vi "fpga_Lowpass filter (P Class_50Hz).vi"(0 "input data":fxp<+/-,24,1>, 1 "reset":bool, 9 "input valid":bool) -> (4 "output data":fxp<+/-,24,2>, 10 "output valid":bool, 14 "ready for input":bool)   [LabVIEW 2013, in "NI_EP_PMU_FPGA.lvlib"]
doc: "----------------------\n\nThis filter is configured as follows:\n\n<b>Filter Configuration</b>\nType: Multirate - Decimation\nStructure: Polyphase FIR\nFactor: 25\n\n<b>Input Data Type</b>\nType: fixed-point <±,24,1> [-1.000000E+0,9.999999E-1]:1.192093E-7\n\n<b>Output Data Type</b>\nType: fixed-point <±,24,2> [-2.000000E+0,2.000000E+0]:2.384186E-7\nRounding mode: Truncate\nOverflow mode: Saturate\n\n<b>Implementation</b>\nNumber of channels: 1\nMaximum input sampling rate per channel @ 40MHz: 8MHz\nGain processing: On Host\nMethod: Multiply-Accumulate\nNumber of multiply pipeline stages: 1\nMultiply register in: False\nState memory: Look-Up Table\nCoefficient memory: Block Memory\n\n<b>Execution Mode</b>\nInside single-cycle Timed Loop\nThroughput: 5 cycles/sample\n\n<b>Estimated Resources</b>\nNumber of multiply-accumulate units: 1\nMultiply operation: I24.1 x I16.-4 => I44.1"
uses:
  <vilib>/addons/Electrical Power/PMU/NI_EP_PMU_FPGA.lvlib
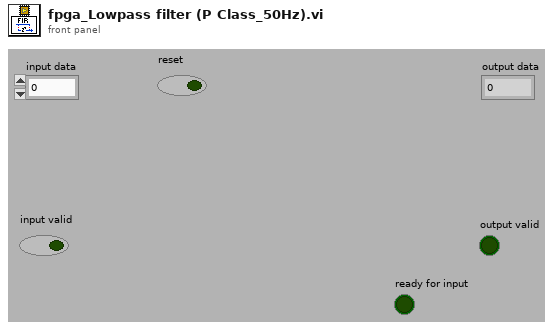
[diagram p1: front panel]
types:
  T1 = cluster{"WRSel":bool, "WREn":bool, "stateMemRDAddr":fxp<+,3,3>, "stateMemWRAddr":fxp<+,3,3>, "firstRun":bool}
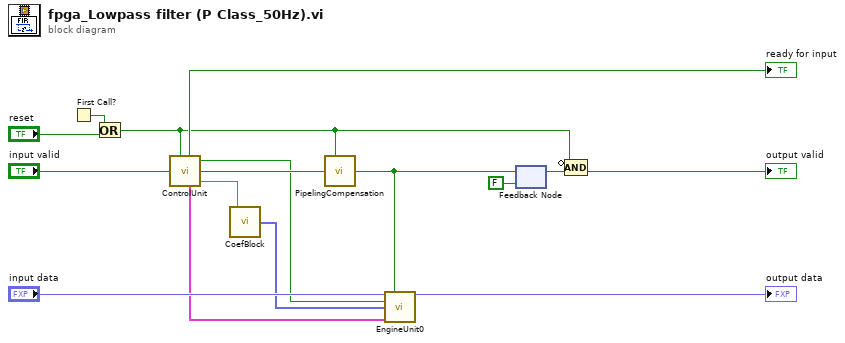
[diagram p0: block diagram]
diagram:
  n1 = First Call?() -> (First Call?: T/F=w11:bool)
  n2 = Or(x=w11, y="reset") -> (x .or. y?=w9:bool)
  n3 = call "ControlUnit"("reset"=w9, "input valid"="input valid") -> ("ready for input"=→"ready for input":bool, "procInputValid"=w6:bool, "output valid"=w13:bool, "opState"=w3:T1, "coefRDAddr"=w8:fxp<+,7,7>)  [unwired: 3 in]
  n4 = call "CoefBlock"("coefAddr"=w8) -> ("coefficients"=w4:fxp<+/-,16,-4>[])  [unwired: 8 in]
  n5 = call "PipelingCompensation"("reset"=w9, "data in"=w13) -> ("data out"=w5:bool)  [unwired: 7 in]
  n6 = call "EngineUnit0"("input data"="input data", "Output_Latch"=w5, "Input_Latch"=w6, "coefficients"=w4, "opState"=w3) -> ("output data"=→"output data":fxp<+/-,24,2>)  [unwired: 10 in]
  n7 = feedback-in #1(w5) -> ()
  n8 = feedback #1(FALSE ("procInputValid")) -> (w14:bool)
  n9 = Compound Arithmetic op=AND(invert w9, w14) -> (→"output valid":bool)
